vi "LM120-5.0.vi"() -> ()   [LabVIEW 2014]
uses:
  tmp/Keithley 24XX/Keithley 24XX.lvlib
panel:
  out "Vout2":dbl[](array[numeric])
  out "Vout1":dbl[](array[numeric])
  out "Iq":dbl[](array[numeric])
  in  "VISA Keythley 2410 - Out":refnum<visa-resource-name>
  in  "Serial Configuration 5":T1={"Baud Rate"=9600, "Parity"=0, "Data Bits"=8, "Stop Bits"=10, "Flow Control"=0} {"Flow Control" items=["None", "XON/XOFF", "RTS/CTS", "XON/XOFF & RTS/CTS", "DTR/DSR", "XON/XOFF & DTR/DSR"]; "Stop Bits" items=["1.0"=10, "1.5"=15, "2.0"=20]; "Data Bits" items=["7"=7, "8"=8]; "Parity" items=["None", "Odd", "Even", "Mark", "Space"]; "Baud Rate" items=["300"=300, "600"=600, "1200"=1200, "2400"=2400, "4800"=4800, "9600"=9600, "19200"=19200]}
  in  "VISA Keythley 2410 - In":refnum<visa-resource-name>
  # "Power supply"
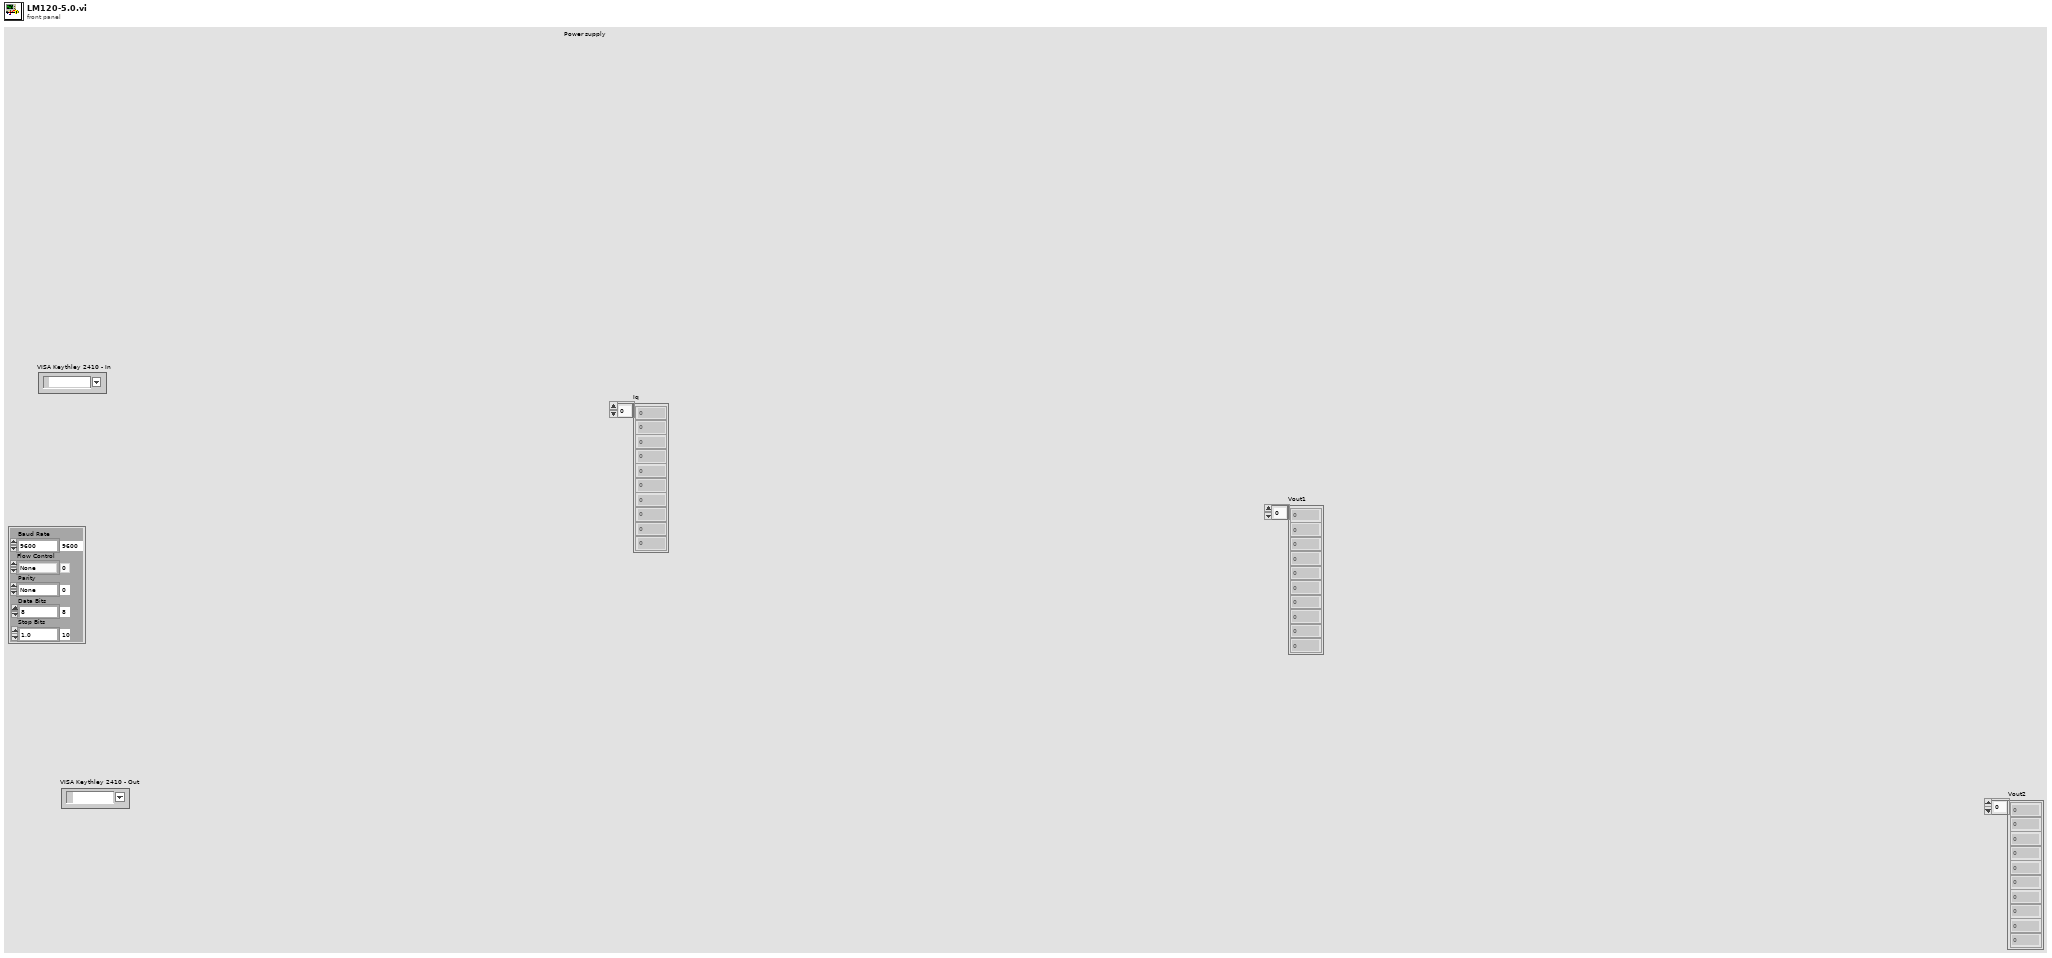
[diagram p1: front panel]
types:
  T1 = cluster{"Baud Rate":u32, "Parity":u16, "Data Bits":u16, "Stop Bits":u16, "Flow Control":u16}
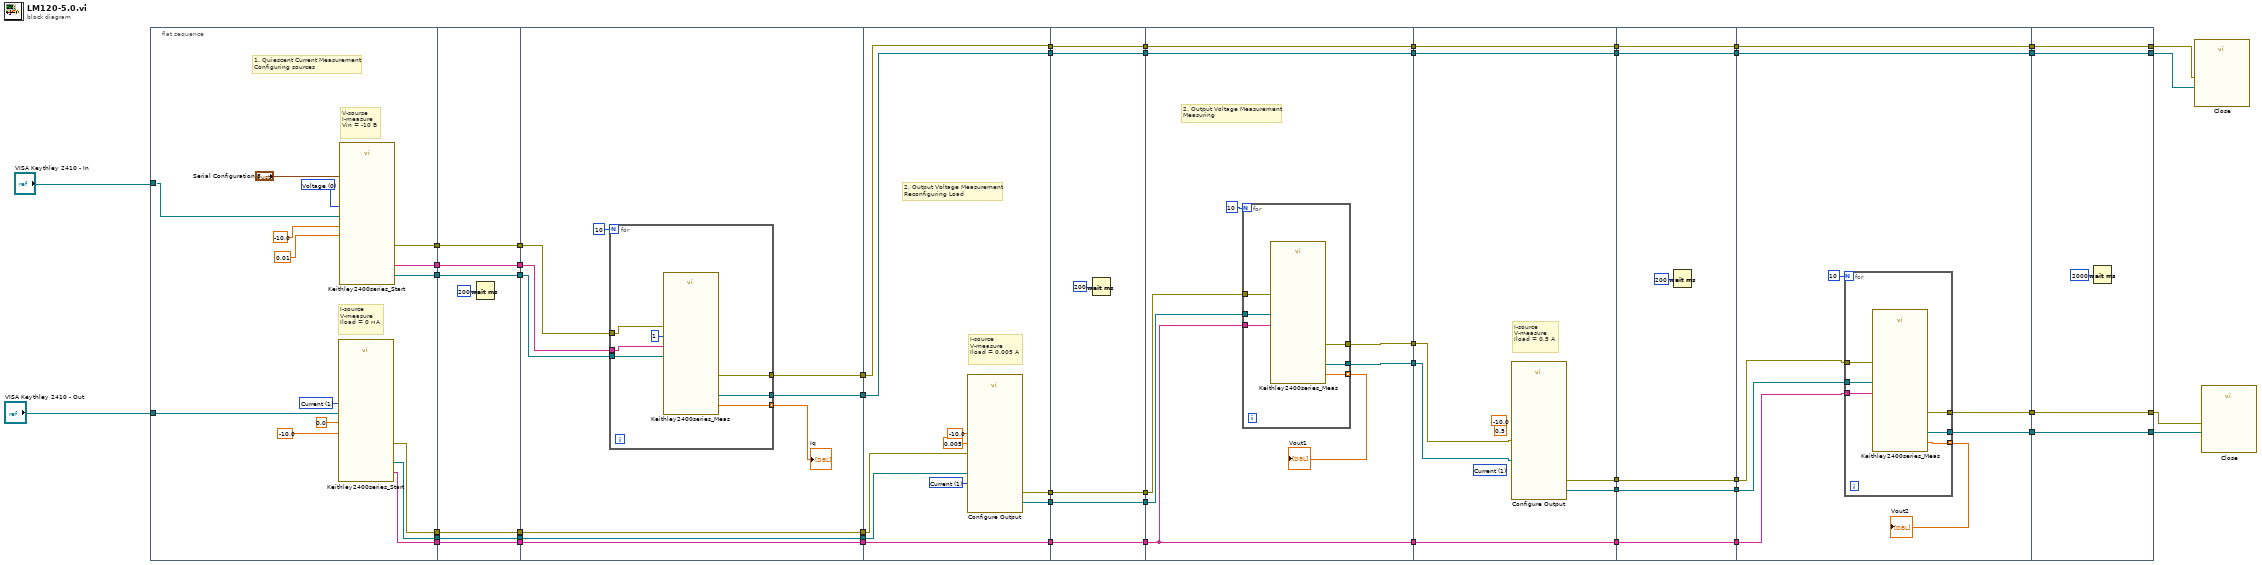
[diagram p0: block diagram]
diagram:
  n1 = flat-sequence {
    tunnel: "VISA Keythley 2410 - In" -> [w63]
    tunnel: "VISA Keythley 2410 - Out" -> [w59]
    tunnel: [w58] -> w50
    tunnel: [w57] -> w49
    tunnel: [w56] -> w48
    tunnel: [w55] -> w42
    tunnel: [w54] -> w41
    tunnel: [w53] -> w40
    tunnel: w50 -> [w73]
    tunnel: w49 -> [w72]
    tunnel: w48 -> [w71]
    tunnel: [w73] -> w47
    tunnel: [w72] -> w46
    tunnel: [w71] -> w45
    tunnel: w42 -> [w68]
    tunnel: w41 -> [w69]
    tunnel: w40 -> [w70]
    tunnel: [w70] -> w39
    tunnel: [w69] -> w38
    tunnel: [w68] -> w37
    tunnel: w47 -> [w80]
    tunnel: w46 -> [w81]
    tunnel: w45 -> [w82]
    tunnel: [w79] -> w44
    tunnel: [w78] -> w43
    tunnel: w39 -> [w77]
    tunnel: w38 -> [w76]
    tunnel: w37 -> [w75]
    tunnel: [w77] -> w36
    tunnel: [w76] -> w35
    tunnel: [w75] -> w34
    tunnel: w44 -> [w93]
    tunnel: w43 -> [w92]
    tunnel: w36 -> [w98]
    tunnel: w35 -> [w97]
    tunnel: w34 -> [w94]
    tunnel: [w96] -> w33
    tunnel: [w95] -> w32
    tunnel: [w94] -> w29
    tunnel: [w93] -> w27
    tunnel: [w92] -> w26
    tunnel: w33 -> [w107]
    tunnel: w32 -> [w106]
    tunnel: [w107] -> w31
    tunnel: [w106] -> w30
    tunnel: w29 -> [w104]
    tunnel: [w104] -> w28
    tunnel: w27 -> [w103]
    tunnel: w26 -> [w102]
    tunnel: [w103] -> w25
    tunnel: [w102] -> w24
    tunnel: w31 -> [w114]
    tunnel: w30 -> [w113]
    tunnel: w28 -> [w108]
    tunnel: w25 -> [w112]
    tunnel: w24 -> [w111]
    tunnel: [w112] -> w23
    tunnel: [w111] -> w22
    tunnel: [w110] -> w21
    tunnel: [w109] -> w20
    tunnel: [w108] -> w19
    tunnel: w23 -> [w129]
    tunnel: w22 -> [w128]
    tunnel: w21 -> [w127]
    tunnel: w20 -> [w126]
    tunnel: w19 -> [w123]
    tunnel: [w129] -> w18
    tunnel: [w128] -> w17
    tunnel: [w125] -> w16
    tunnel: [w124] -> w15
    tunnel: [w123] -> w14
    tunnel: w18 -> [w135]
    tunnel: w17 -> [w134]
    tunnel: w16 -> [w130]
    tunnel: w15 -> [w131]
    tunnel: w14 -> [w132]
    tunnel: [w135] -> w13
    tunnel: [w134] -> w12
    tunnel: [w132] -> w11
    tunnel: [w131] -> w10
    tunnel: [w130] -> w9
    tunnel: w13 -> [w144]
    tunnel: w12 -> [w143]
    tunnel: w11 -> [w138]
    tunnel: w10 -> [w139]
    tunnel: w9 -> [w140]
    tunnel: [w144] -> w8
    tunnel: [w143] -> w7
    tunnel: [w137] -> w6
    tunnel: [w136] -> w5
    tunnel: [w152] -> w1
    tunnel: [w153] -> w2
    tunnel: [w154] -> w3
    tunnel: [w155] -> w4
    tunnel: w8 -> [w155]
    tunnel: w7 -> [w154]
    tunnel: w6 -> [w153]
    tunnel: w5 -> [w152]
    frame #0 {
      w60 = u16 1 items=["Voltage", "Current"] ("Source Mode  (0: Voltage) 2")
      w66 = u16 0 items=["Voltage", "Current"] ("Source Mode  (0: Voltage) 2")
      # "1. Quiescent Current Measurement\nConfiguring sources"
      # "I-source\nV-measure\nIload = 0 мА"
      # "V-sourse\nI-measure\nVin = -10 В"
      n2 = call "Keithley2400series_Start.vi"("Source Mode  (0: Voltage) 2"=w60, "Ограничение"=-10.0 ("Compliance  Level (0.1)"), "Выход"=0.0 ("Output Level (0)"), "VISA resource name"=w59) -> ("error out"=w53:errorcluster, "MEAS:Out"=w55:string, "VISA resource name out"=w54:refnum<visa-resource-name>)  [unwired: 1 in, 1 out]
      n3 = call "Keithley2400series_Start.vi"("Serial Configuration"="Serial Configuration 5", "Source Mode  (0: Voltage) 2"=w66, "Ограничение"=0.01, "Выход"=-10.0, "VISA resource name"=w63) -> ("error out"=w58:errorcluster, "MEAS:Out"=w57:string, "VISA resource name out"=w56:refnum<visa-resource-name>)  [unwired: 1 out]
    }
    frame #1 {
      n4 = Wait (ms)(milliseconds to wait=u32 200) -> ()  [unwired: 1 out]
    }
    frame #2 {
      n5 = for {
        N: 10 -> [_]
        tunnel: [w91] -> w84 mode=indexing
        tunnel: [w90] -> w78
        tunnel: [w89] -> w79
        tunnel: w82 -> [w87]
        tunnel: w81 -> [w86]
        tunnel: w80 -> [w85]
        n6 = call "Keithley2400series_Meas.vi"("MEAS:<f>"=w86, "error in (no error)"=w85, "MEAS mode, 0 Volt"=u16 1, "VISA resource name in"=w87) -> ("error out"=w89:errorcluster, "Замер"=w91:dbl, "VISA out"=w90:refnum<visa-resource-name>)  [unwired: 1 in, 1 out]
      }
      "Iq" <- w84
    }
    frame #3 {
      w101 = u16 1 items=["Voltage", "Current"] ("Source Mode  (0: Voltage)")
      # "2. Output Voltage Measurement\nReconfiguring Load"
      # "I-source\nV-measure\nIload = 0.005 А"
      n7 = call "Configure Output.vi"("Source Mode  (0: Voltage)"=w101, "error in (no error)"=w98, "Compliance  Level (0.1)"=-10.0, "Output Level (0)"=0.005, "VISA resource name"=w97) -> ("error out"=w96:errorcluster, "VISA resource name out"=w95:refnum<visa-resource-name>)  [unwired: 5 in]
    }
    frame #4 {
      n8 = Wait (ms)(milliseconds to wait=u32 200) -> ()  [unwired: 1 out]
    }
    frame #5 {
      # "2. Output Voltage Measurement\nMeasuring"
      n9 = for {
        N: 10 -> [_]
        tunnel: [w122] -> w115 mode=indexing
        tunnel: w114 -> [w121]
        tunnel: w113 -> [w120]
        tunnel: w108 -> [w119]
        tunnel: [w118] -> w110
        tunnel: [w117] -> w109
        n10 = call "Keithley2400series_Meas.vi"("MEAS:<f>"=w119, "error in (no error)"=w121, "VISA resource name in"=w120) -> ("error out"=w117:errorcluster, "Замер"=w122:dbl, "VISA out"=w118:refnum<visa-resource-name>)  [unwired: 2 in, 1 out]
      }
      "Vout1" <- w115
    }
    frame #6 {
      (unwired) -10.0 ("Compliance  Level (0.1)")
      (unwired) 0.5 ("Output Level (0)")
      (unwired) u16 1 items=["Voltage", "Current"] ("Source Mode  (0: Voltage)")
      # "I-source\nV-measure\nIload = 0.5 А"
      n11 = call "Configure Output.vi"("error in (no error)"=w126, "VISA resource name"=w127) -> ("error out"=w125:errorcluster, "VISA resource name out"=w124:refnum<visa-resource-name>)  [unwired: 8 in]
    }
    frame #7 {
      n12 = Wait (ms)(milliseconds to wait=u32 200) -> ()  [unwired: 1 out]
    }
    frame #8 {
      n13 = for {
        N: 10 -> [_]
        tunnel: [w150] -> w141 mode=indexing
        tunnel: w140 -> [w149]
        tunnel: w139 -> [w148]
        tunnel: w138 -> [w147]
        tunnel: [w146] -> w136
        tunnel: [w145] -> w137
        n14 = call "Keithley2400series_Meas.vi"("MEAS:<f>"=w147, "error in (no error)"=w149, "VISA resource name in"=w148) -> ("error out"=w145:errorcluster, "Замер"=w150:dbl, "VISA out"=w146:refnum<visa-resource-name>)  [unwired: 2 in, 1 out]
      }
      "Vout2" <- w141
    }
    frame #9 {
      n15 = Wait (ms)(milliseconds to wait=u32 2000) -> ()  [unwired: 1 out]
    }
  }
  n16 = call "Close.vi"("error in (no error)"=w4, "VISA resource name"=w3) -> ()  [unwired: 9 in, 1 out]
  n17 = call "Close.vi"("error in (no error)"=w2, "VISA resource name"=w1) -> ()  [unwired: 9 in, 1 out]
